vi "Plane offset string.vi"() -> ()   [LabVIEW 2014]
panel:
  in  "Z":dbl
  in  "Y":dbl
  in  "X":dbl
  in  "String in":string
  out "ProgramList out":string[](array[string])
  in  "ProgramList in":string[](array[string])
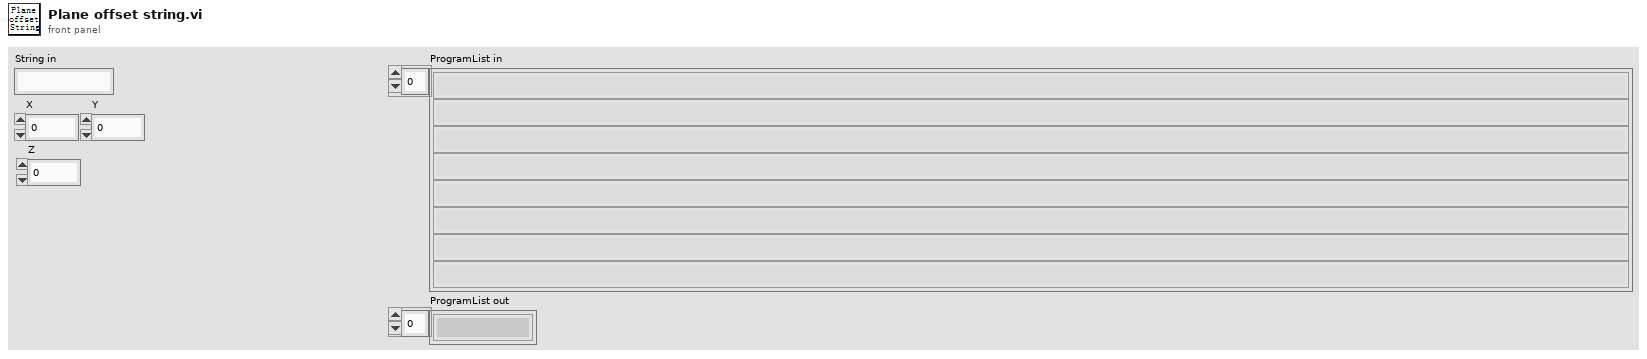
[diagram p1: front panel]
types:
  T1 = cluster{"X":dbl, "Y":dbl, "Z":dbl, "R":dbl, "T":dbl}
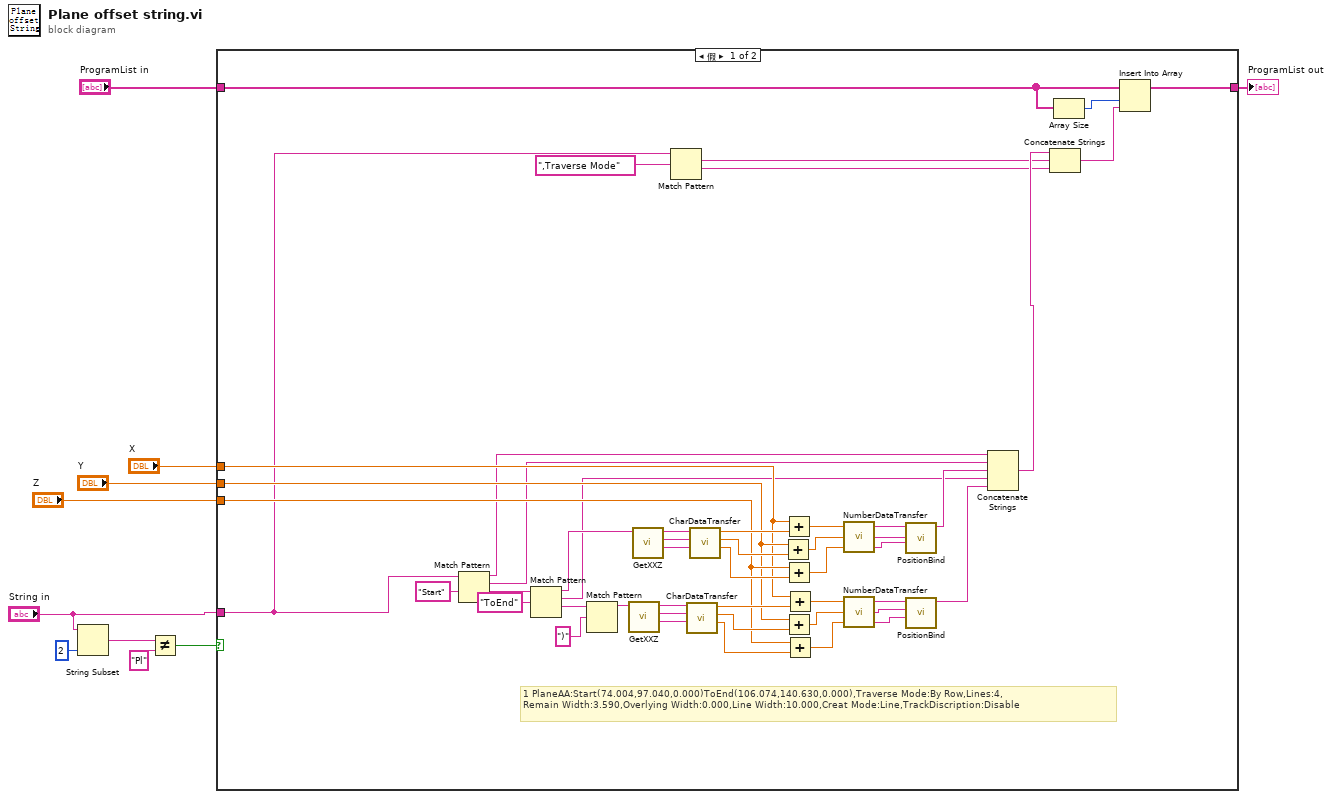
[diagram p0: block diagram]
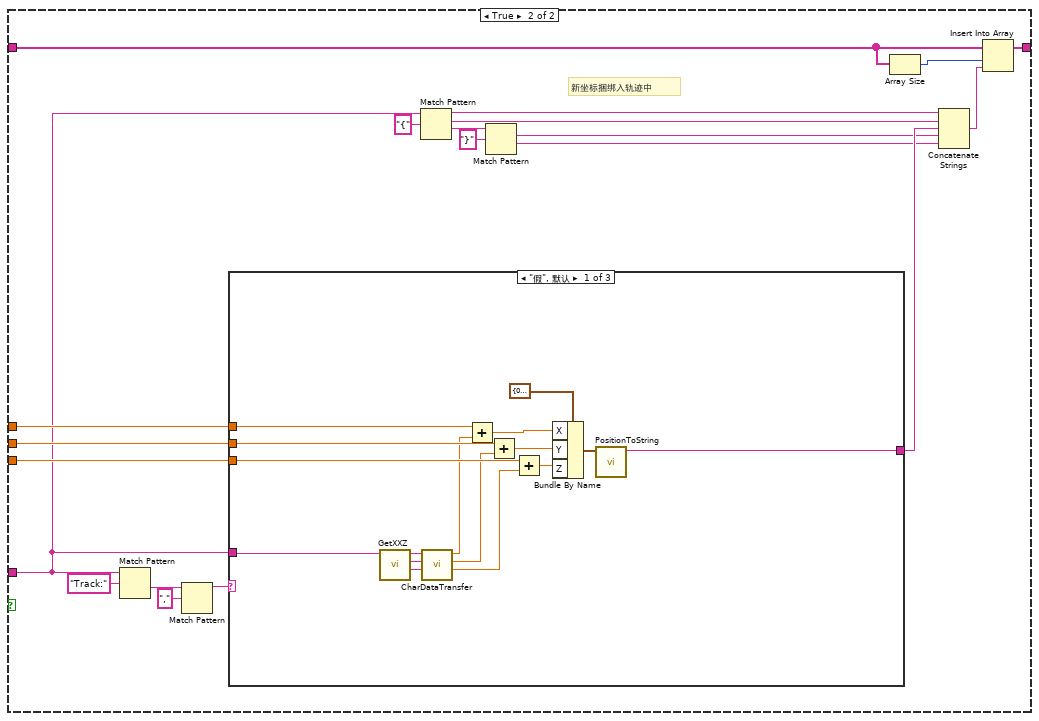
[diagram p2: hidden frame]
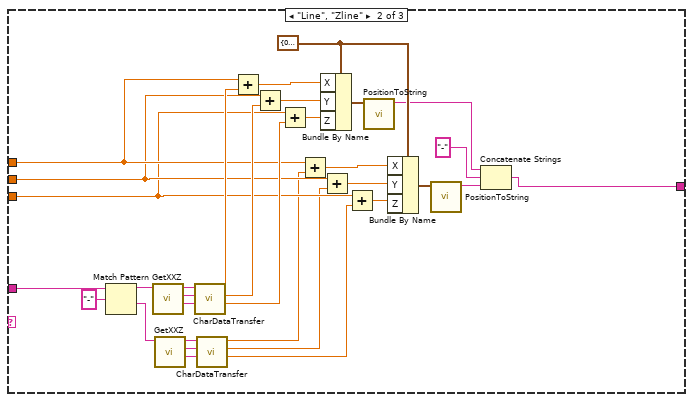
[diagram p3: hidden frame]
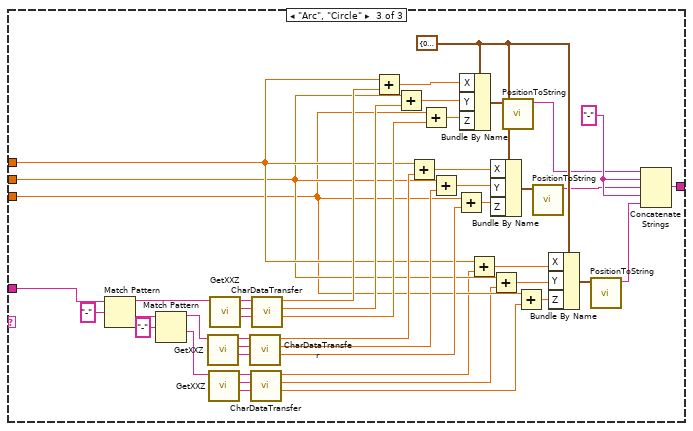
[diagram p4: hidden frame]
diagram:
  n1 = String Subset(string="String in", length (rest)=2 ("长度（剩余）")) -> (substring=w2:string)  [unwired: 1 in]
  n2 = Not Equal?(x=w2, y="Pl") -> (x != y?=w1:bool)
  n3 = case shown="假" w1 {
    tunnel: "X" -> [w37 w78]
    tunnel: "Y" -> [w38 w77]
    tunnel: "Z" -> [w39 w76]
    tunnel: "ProgramList in" -> [w13 w65]
    tunnel: [w14 w71] -> w9
    tunnel: "String in" -> [w11 w59]
    frame False {
      # "1 PlaneAA:Start(74.004,97.040,0.000)ToEnd(106.074,140.630,0.000),Traverse Mode:By Row,Lines:4,\nRemain Width:3.590,Overlying Width:0.000,Line Width:10.000,Creat Mode:Line,TrackDiscription:Disable"
      n4 = Match Pattern(string=w11, regular expression="Start" ("正则表达式")) -> (before substring=w24:string, match substring=w23:string, after substring=w57:string)  [unwired: 1 in, 1 out]
      n5 = Match Pattern(string=w57, regular expression="ToEnd" ("正则表达式")) -> (before substring=w53:string, match substring=w21:string, after substring=w55:string)  [unwired: 1 in, 1 out]
      n6 = Match Pattern(string=w55, regular expression=")" ("正则表达式")) -> (before substring=w52:string)  [unwired: 1 in, 3 out]
      n7 = call "GetXXZ.vi"("TrackIn"=w52) -> ("Z"=w43:string, "Y"=w44:string, "X"=w45:string)  [unwired: 6 in, 2 out]
      n8 = call "GetXXZ.vi"("TrackIn"=w53) -> ("Z"=w49:string, "Y"=w50:string, "X"=w51:string)  [unwired: 6 in, 2 out]
      n9 = Match Pattern(string=w11, regular expression=",Traverse Mode") -> (match substring=w17:string, after substring=w16:string)  [unwired: 1 in, 2 out]
      n10 = call "CharDataTransfer.vi"("Z"=w43, "Y"=w44, "X"=w45) -> ("Z"=w40:dbl, "Y"=w41:dbl, "X"=w42:dbl)  [unwired: 1 in, 1 out]
      n11 = call "CharDataTransfer.vi"("Z"=w49, "Y"=w50, "X"=w51) -> ("Z"=w46:dbl, "Y"=w48:dbl, "X"=w47:dbl)  [unwired: 1 in, 1 out]
      n12 = Add(x=w38, y=w48) -> (x+y=w35:dbl)
      n13 = Add(x=w37, y=w47) -> (x+y=w36:dbl)
      n14 = Add(x=w39, y=w46) -> (x+y=w34:dbl)
      n15 = Add(x=w38, y=w41) -> (x+y=w32:dbl)
      n16 = Add(x=w37, y=w42) -> (x+y=w33:dbl)
      n17 = Add(x=w39, y=w40) -> (x+y=w31:dbl)
      n18 = call "NumberDataTransfer.vi"("Z"=w34, "Y"=w35, "X"=w36) -> ("Z"=w28:string, "Y"=w29:string, "X"=w30:string)
      n19 = call "NumberDataTransfer.vi"("Z"=w31, "Y"=w32, "X"=w33) -> ("Z"=w25:string, "Y"=w26:string, "X"=w27:string)
      n20 = call "PositionBind.vi"("Z"=w28, "Y"=w29, "X"=w30) -> ("PosOut"=w22:string)  [unwired: 8 in]
      n21 = call "PositionBind.vi"("Z"=w25, "Y"=w26, "X"=w27) -> ("PosOut"=w20:string)  [unwired: 8 in]
      n22 = Concatenate Strings(w24, w23, w22, w21, w20) -> (w18:string)
      n23 = Concatenate Strings(w18, w17, w16) -> (w15:string)
      n24 = Array Size(array=w13) -> (size(s)=w12:i32)
      n25 = Insert Into Array(array=w13, index=w12, new element=w15) -> (w14:string[])
    }
    frame True {
      # "新坐标捆绑入轨迹中"
      n26 = Match Pattern(string=w59, regular expression="Track:" ("正则表达式")) -> (after substring=w61:string)  [unwired: 1 in, 3 out]
      n27 = Match Pattern(string=w61, regular expression="," ("正则表达式")) -> (before substring=w60:string)  [unwired: 1 in, 3 out]
      n28 = case shown="\"假\", 默认" w60 {
        tunnel: w59 -> [w79 w95 w127]
        tunnel: w78 -> [w91 w106 w141]
        tunnel: w77 -> [w90 w105 w140]
        tunnel: w76 -> [w89 w104 w139]
        tunnel: [w80 w99 w129] -> w70
        frame "假", Default {
          n29 = call "GetXXZ.vi"("TrackIn"=w79) -> ("Z"=w93:string, "Y"=w94:string, "X"=w92:string)  [unwired: 6 in, 2 out]
          n30 = call "CharDataTransfer.vi"("Z"=w93, "Y"=w94, "X"=w92) -> ("Z"=w86:dbl, "Y"=w87:dbl, "X"=w88:dbl)  [unwired: 1 in, 1 out]
          n31 = Add(x=w91, y=w88) -> (x+y=w84:dbl)
          n32 = Add(x=w90, y=w87) -> (x+y=w83:dbl)
          n33 = Add(x=w89, y=w86) -> (x+y=w82:dbl)
          n34 = Bundle By Name(cluster=T1 {"X"=0.0, "Y"=0.0, "Z"=0.0, "R"=0.0, "T"=0.0} ("Position"), "X"=w84, "Y"=w83, "Z"=w82) -> (w81:T1)
          n35 = call "PositionToString.vi"("Position"=w81) -> ("Position"=w80:string)  [unwired: 7 in, 3 out]
        }
        frame "Line", "Zline" {
          w100 = T1 {"X"=0.0, "Y"=0.0, "Z"=0.0, "R"=0.0, "T"=0.0} ("Position")
          n36 = Match Pattern(string=w95, regular expression="-" ("正则表达式")) -> (before substring=w122:string, after substring=w118:string)  [unwired: 1 in, 2 out]
          n37 = call "GetXXZ.vi"("TrackIn"=w122) -> ("Z"=w124:string, "Y"=w125:string, "X"=w123:string)  [unwired: 6 in, 2 out]
          n38 = call "GetXXZ.vi"("TrackIn"=w118) -> ("Z"=w120:string, "Y"=w119:string, "X"=w121:string)  [unwired: 6 in, 2 out]
          n39 = call "CharDataTransfer.vi"("Z"=w124, "Y"=w125, "X"=w123) -> ("Z"=w111:dbl, "Y"=w112:dbl, "X"=w113:dbl)  [unwired: 1 in, 1 out]
          n40 = call "CharDataTransfer.vi"("Z"=w120, "Y"=w119, "X"=w121) -> ("Z"=w101:dbl, "Y"=w102:dbl, "X"=w103:dbl)  [unwired: 1 in, 1 out]
          n41 = Add(x=w106, y=w113) -> (x+y=w117:dbl)
          n42 = Add(x=w105, y=w112) -> (x+y=w116:dbl)
          n43 = Add(x=w104, y=w111) -> (x+y=w115:dbl)
          n44 = Add(x=w106, y=w103) -> (x+y=w107:dbl)
          n45 = Bundle By Name(cluster=w100, "X"=w117, "Y"=w116, "Z"=w115) -> (w114:T1)
          n46 = Add(x=w105, y=w102) -> (x+y=w108:dbl)
          n47 = Add(x=w104, y=w101) -> (x+y=w109:dbl)
          n48 = call "PositionToString.vi"("Position"=w114) -> ("Position"=w98:string)  [unwired: 7 in, 3 out]
          n49 = Bundle By Name(cluster=w100, "X"=w107, "Y"=w108, "Z"=w109) -> (w110:T1)
          n50 = call "PositionToString.vi"("Position"=w110) -> ("Position"=w97:string)  [unwired: 7 in, 3 out]
          n51 = Concatenate Strings(w98, "-" ("字符串"), w97) -> (w99:string)
        }
        frame "Arc", "Circle" {
          w132 = "-" ("字符串")
          w142 = T1 {"X"=0.0, "Y"=0.0, "Z"=0.0, "R"=0.0, "T"=0.0} ("Position")
          n52 = Match Pattern(string=w127, regular expression="-" ("正则表达式")) -> (before substring=w166:string, after substring=w170:string)  [unwired: 1 in, 2 out]
          n53 = Match Pattern(string=w170, regular expression="-" ("正则表达式")) -> (before substring=w162:string, after substring=w158:string)  [unwired: 1 in, 2 out]
          n54 = call "GetXXZ.vi"("TrackIn"=w162) -> ("Z"=w164:string, "Y"=w163:string, "X"=w165:string)  [unwired: 6 in, 2 out]
          n55 = call "GetXXZ.vi"("TrackIn"=w158) -> ("Z"=w160:string, "Y"=w161:string, "X"=w159:string)  [unwired: 6 in, 2 out]
          n56 = call "GetXXZ.vi"("TrackIn"=w166) -> ("Z"=w168:string, "Y"=w169:string, "X"=w167:string)  [unwired: 6 in, 2 out]
          n57 = call "CharDataTransfer.vi"("Z"=w164, "Y"=w163, "X"=w165) -> ("Z"=w147:dbl, "Y"=w148:dbl, "X"=w149:dbl)  [unwired: 1 in, 1 out]
          n58 = call "CharDataTransfer.vi"("Z"=w160, "Y"=w161, "X"=w159) -> ("Z"=w133:dbl, "Y"=w134:dbl, "X"=w135:dbl)  [unwired: 1 in, 1 out]
          n59 = call "CharDataTransfer.vi"("Z"=w168, "Y"=w169, "X"=w167) -> ("Z"=w151:dbl, "Y"=w152:dbl, "X"=w153:dbl)  [unwired: 1 in, 1 out]
          n60 = Add(x=w141, y=w153) -> (x+y=w157:dbl)
          n61 = Add(x=w140, y=w152) -> (x+y=w156:dbl)
          n62 = Add(x=w141, y=w149) -> (x+y=w146:dbl)
          n63 = Add(x=w139, y=w151) -> (x+y=w155:dbl)
          n64 = Add(x=w140, y=w148) -> (x+y=w145:dbl)
          n65 = Add(x=w139, y=w147) -> (x+y=w144:dbl)
          n66 = Bundle By Name(cluster=w142, "X"=w157, "Y"=w156, "Z"=w155) -> (w154:T1)
          n67 = Add(x=w141, y=w135) -> (x+y=w138:dbl)
          n68 = Bundle By Name(cluster=w142, "X"=w146, "Y"=w145, "Z"=w144) -> (w150:T1)
          n69 = Add(x=w140, y=w134) -> (x+y=w137:dbl)
          n70 = call "PositionToString.vi"("Position"=w154) -> ("Position"=w131:string)  [unwired: 7 in, 3 out]
          n71 = Add(x=w139, y=w133) -> (x+y=w136:dbl)
          n72 = call "PositionToString.vi"("Position"=w150) -> ("Position"=w130:string)  [unwired: 7 in, 3 out]
          n73 = Bundle By Name(cluster=w142, "X"=w138, "Y"=w137, "Z"=w136) -> (w143:T1)
          n74 = call "PositionToString.vi"("Position"=w143) -> ("Position"=w128:string)  [unwired: 7 in, 3 out]
          n75 = Concatenate Strings(w131, w132, w130, w132, w128) -> (w129:string)
        }
      }
      n76 = Match Pattern(string=w59, regular expression="{" ("正则表达式")) -> (before substring=w69:string, match substring=w68:string, after substring=w74:string)  [unwired: 1 in, 1 out]
      n77 = Match Pattern(string=w74, regular expression="}" ("正则表达式")) -> (match substring=w67:string, after substring=w66:string)  [unwired: 1 in, 2 out]
      n78 = Array Size(array=w65) -> (size(s)=w64:i32)
      n79 = Concatenate Strings(w69, w68, w70, w67, w66) -> (w72:string)
      n80 = Insert Into Array(array=w65, index=w64, new element=w72) -> (w71:string[])
    }
  }
  "ProgramList out" <- w9
